vi "UpdateChannelWiringStatus.vi"(8 "error in (no error)":errorcluster, 10 "Waveforms In":waveform(sgl)[](array[waveform]), 11 "Group":T1) -> (0 "error out":errorcluster, 2 "Waveforms Out":waveform(sgl)[](array[waveform]), 3 "Group out":T1)   [LabVIEW 2017, in "McsaAnalysisLowRate.lvlib"]
uses:
  <vilib>/addons/InsightCM/Devices/Shared/Mcsa/McsaAnalysisLowRate/McsaAnalysisLowRate.lvlib
  <vilib>/addons/InsightCM/Devices/Shared/Mcsa/McsaAnalysisLowRate/controls/Group.ctl
  <vilib>/addons/InsightCM/Utilities/Analysis/MCSA/controls/McsaChannel.ctl
  <vilib>/addons/InsightCM/Utilities/Analysis/Shared/controls/Feature.ctl
  <vilib>/addons/InsightCM/Utilities/Analysis/Shared/controls/AmplitudeScale.ctl
  <vilib>/addons/InsightCM/MessageBus/Base/controls/KeyValuePair.ctl
  <vilib>/addons/InsightCM/Utilities/Analysis/MCSA/controls/McsaChannelPhasor.ctl
  <vilib>/addons/InsightCM/Utilities/Analysis/MCSA/controls/McsaMotor.ctl
  <vilib>/addons/InsightCM/Utilities/Analysis/MCSA/controls/MotorCalculationCache.ctl
  <vilib>/addons/Electrical Power/Basic/Measurement/subVIs/basic_Power Value.ctl
  <vilib>/addons/InsightCM/Utilities/Analysis/MCSA/controls/TorqueLoadEfficiency.ctl
  <vilib>/addons/InsightCM/Utilities/Analysis/Shared/AnalysisHelper.lvlib
  <vilib>/addons/InsightCM/Utilities/Analysis/MCSA/McsaAnalysisFunctions.lvlib
  <vilib>/addons/Electrical Power/Basic/NI_EP_Basic.lvlib
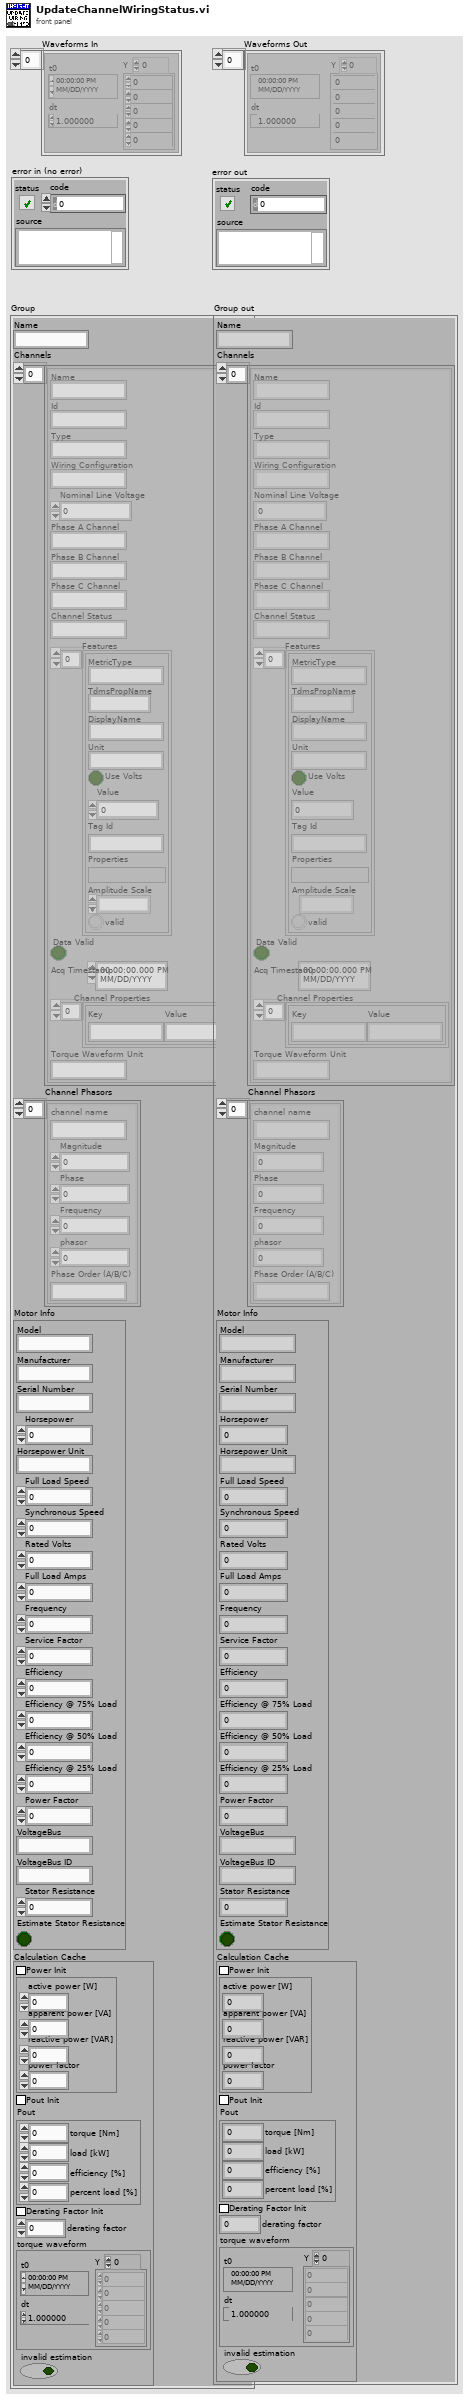
[diagram p1: front panel]
types:
  T1 = typedef "McsaAnalysisLowRate.lvlib/Group.ctl" = cluster{"Name":string, "Channels":T2[], "Channel Phasors":T6[], "Motor Info":T7, "Calculation Cache":T8}
  T2 = typedef "McsaAnalysisFunctions.lvlib/McsaChannel.ctl" = cluster{"Name":string, "Id":string, "Type":string, "Wiring Configuration":string, "Nominal Line Voltage":dbl, "Phase A Channel":string, "Phase B Channel":string, "Phase C Channel":string, "Channel Status":string, "Features":T3[], "Data Valid":bool, "Acq Timestamp":timestamp, "Channel Properties":T5[], "Torque Waveform Unit":string}
  T3 = typedef "AnalysisHelper.lvlib/Feature.ctl" = cluster{"MetricType":string, "TdmsPropName":string, "DisplayName":string, "Unit":string, "Use Volts":bool, "Value":dbl, "Tag Id":string, "Properties":variant, "Amplitude Scale":T4, "valid":bool}
  T4 = typedef "AnalysisHelper.lvlib/AmplitudeScale.ctl" = enum16{"rms", "peak", "pk-pk"}
  T5 = typedef "KeyValuePair.ctl" = cluster{"Key":string, "Value":string}
  T6 = typedef "McsaAnalysisFunctions.lvlib/McsaChannelPhasor.ctl" = cluster{"channel name":string, "Magnitude":dbl, "Phase":dbl, "Frequency":dbl, "phasor":cdb, "Phase Order (A/B/C)":string}
  T7 = typedef "McsaAnalysisFunctions.lvlib/McsaMotor.ctl" = cluster{"Model":string, "Manufacturer":string, "Serial Number":string, "Horsepower":dbl, "Horsepower Unit":string, "Full Load Speed":dbl, "Synchronous Speed":dbl, "Rated Volts":dbl, "Full Load Amps":dbl, "Frequency":dbl, "Service Factor":dbl, "Efficiency":dbl, "Efficiency @ 75% Load":dbl, "Efficiency @ 50% Load":dbl, "Efficiency @ 25% Load":dbl, "Power Factor":dbl, "VoltageBus":string, "VoltageBus ID":string, "Stator Resistance":dbl, "Estimate Stator Resistance":bool}
  T8 = typedef "McsaAnalysisFunctions.lvlib/MotorCalculationCache.ctl" = cluster{"Power Init":bool, "power value":T9, "Pout Init":bool, "Pout":T10, "Derating Factor Init":bool, "derating factor":sgl, "torque waveform":waveform(dbl), "invalid estimation":bool}
  T9 = typedef "NI_EP_Basic.lvlib/basic_Power Value.ctl" = cluster{"active power [W]":dbl, "apparent power [VA]":dbl, "reactive power [VAR]":dbl, "power factor":dbl}
  T10 = typedef "McsaAnalysisFunctions.lvlib/TorqueLoadEfficiency.ctl" = cluster{"torque [Nm]":dbl, "load [kW]":dbl, "efficiency [%]":dbl, "percent load [%]":dbl}
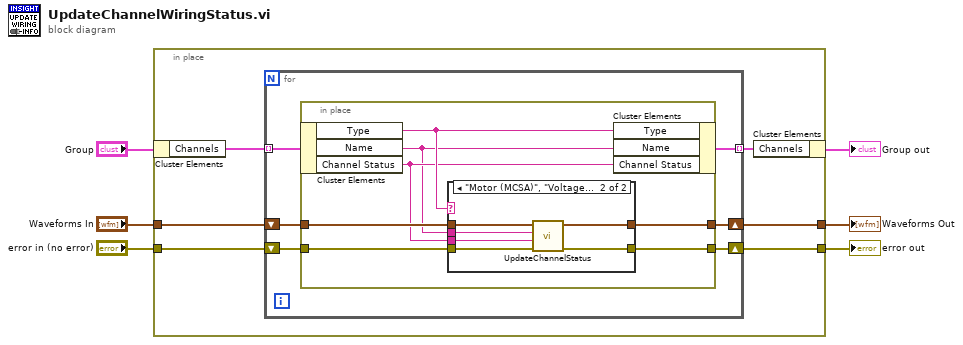
[diagram p0: block diagram]
diagram:
  n1 = in-place {
    in-place-border: "error in (no error)" -> [w9]
    in-place-border: [w10] -> w6
    in-place-border: "Waveforms In" -> [w7]
    in-place-border: [w8] -> w1
    n2 = in-place-cluster #1("Group") -> ("Channels"=w12:T2[])
    n3 = for {
      tunnel: w12 -> [w18] mode=indexing
      tunnel: [w16] -> w11 mode=indexing
      shift-right: [w13] -> w10
      shift-left: w9 -> [w17]
      shift-right: [w15] -> w8
      shift-left: w7 -> [w14]
      n4 = in-place {
        in-place-border: w17 -> [w24]
        in-place-border: w14 -> [w23]
        in-place-border: [w20] -> w15
        in-place-border: [w19] -> w13
        n5 = in-place-cluster #2(w18) -> ("Type"=w25:string, "Name"=w21:string, "Channel Status"=w22:string)
        n6 = case shown="\"Motor (MCSA)\", \"Voltage Bus\"" w25 {
          tunnel: w22 -> [_ w32]
          tunnel: w24 -> [w27 w33]
          tunnel: w23 -> [w26 w31]
          tunnel: w21 -> [_ w30]
          tunnel: [w27 w29] -> w19
          tunnel: [w26 w28] -> w20
          frame Default {
          }
          frame "Motor (MCSA)", "Voltage Bus" {
            n7 = call <vilib>:"UpdateChannelStatus.vi"("error in (no error)"=w33, "Channel Status"=w32, "Channel Name"=w30, "Waveforms in"=w31) -> ("error out"=w29:errorcluster, "Waveforms out"=w28:waveform(sgl)[])  [unwired: 6 in]
          }
        }
        n8 = in-place-cluster #2("Type"=w25, "Name"=w21, "Channel Status"=w22) -> (w16:T2)
      }
    }
    n9 = in-place-cluster #1("Channels"=w11) -> (→"Group out":T1)
  }
  "error out" <- w6
  "Waveforms Out" <- w1
